vi "Scanning Status.vi"(10 "Ready to Scan":bool, 11 "Done out":bool) -> (2 "Next Status":T1(ring))   [LabVIEW 2015]
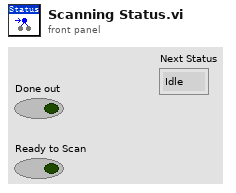
[diagram p1: front panel]
types:
  T1 = enum16{"Idle", "Init", "Write", "Scan", "Blank", "Stop"}
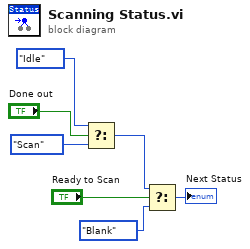
[diagram p0: block diagram]
diagram:
  n1 = Select(t=T1."Idle", s="Done out", f=T1."Scan") -> (s? t:f=w6:T1)
  n2 = Select(t=w6, s="Ready to Scan", f=T1."Blank") -> (s? t:f=→"Next Status":T1)
